vi "Close.vi"(8 "error in (no error)":errorcluster, 10 "write if changed (T)":bool=TRUE, 11 "ODBC-Interface in":refnum<class "ODBC-Interface.lvclass">) -> (0 "error out":errorcluster, 3 "ODBC-Interface out":refnum<class "ODBC-Interface.lvclass">)   [LabVIEW 2014, in "DB-Configuration.lvlib" / "ODBC-Interface.lvclass"]
doc: "Close connection to ODBC database."
uses:
  ODBC-Interface.lvclass
  <vilib>/addons/database/Connection.llb/Conn ObjectReference.ctl
  ODBC-Interface.lvclass/ODBC-Interface.ctl
  <vilib>/addons/database/NI_Database_API.lvlib
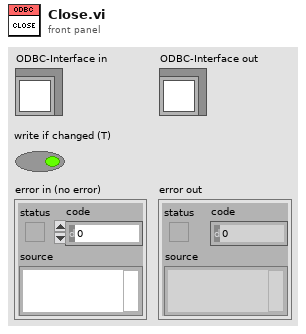
[diagram p1: front panel]
types:
  T1 = typedef "NI_Database_API.lvlib/Conn ObjectReference.ctl" = refnum<k1>
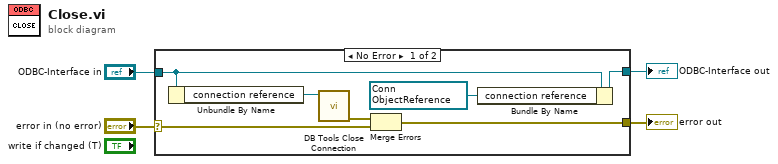
[diagram p0: block diagram]
diagram:
  n1 = case shown="No Error" "error in (no error)" {
    selector: "error in (no error)" -> [w7 w12]
    tunnel: [w6 w12] -> w4
    tunnel: "ODBC-Interface in" -> [w9 w13]
    tunnel: [w8 w13] -> w2
    frame No Error {
      w10 = T1 refnum items=["Connection"] ("connection reference")
      n2 = Unbundle By Name(w9) -> ("connection reference"=w11:T1)
      n3 = call <vilib>:"DB Tools Close Connection.vi"("connection reference"=w11) -> ("error out"=w5:errorcluster)  [unwired: 6 in]
      n4 = Merge Errors(w5, w7) -> (w6:errorcluster)
      n5 = Bundle By Name(cluster=w9, "connection reference"=w10) -> (w8:refnum<class "ODBC-Interface.lvclass">)
    }
    frame Error {
    }
  }
  "error out" <- w4
  "ODBC-Interface out" <- w2
